vi "Write SP.vi"(8 "error in (no error)":errorcluster, 10 "SP":dbl, 11 "Y_H in":refnum<class "Y_H.lvclass">) -> (0 "error out":errorcluster, 3 "Y_H out":refnum<class "Y_H.lvclass">)   [LabVIEW 2019, in "Y_H.lvclass"]
uses:
  Y_H.lvclass
  Y_H.lvclass/Y_H.ctl
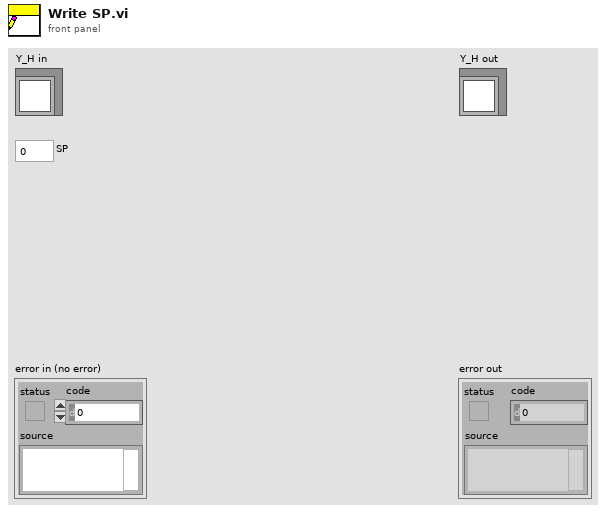
[diagram p1: front panel]
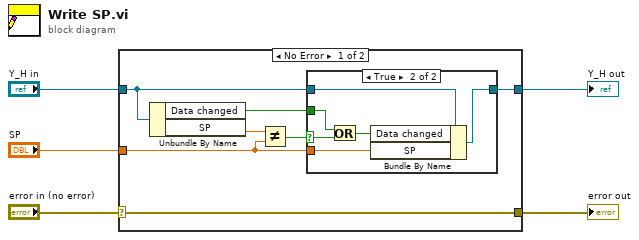
[diagram p0: block diagram]
diagram:
  n1 = case shown="No Error" "error in (no error)" {
    selector: "error in (no error)" -> [w12 w20]
    tunnel: [w12 w20] -> w1
    tunnel: [w11 w21] -> w2
    tunnel: "Y_H in" -> [w10 w21]
    tunnel: "SP" -> [w8 _]
    frame No Error {
      n2 = Unbundle By Name(w10) -> ("Data changed"=w6:bool, "SP"=w9:dbl)
      n3 = Not Equal?(x=w9, y=w8) -> (x != y?=w7:bool)
      n4 = case shown="True" w7 {
        selector: w7 -> [_ w16]
        tunnel: [w13 w19] -> w11
        tunnel: w10 -> [w13 w18]
        tunnel: w8 -> [_ w17]
        tunnel: w6 -> [_ w14]
        frame False {
        }
        frame True {
          n5 = Or(x=w14, y=w16) -> (x .or. y?=w15:bool)
          n6 = Bundle By Name(cluster=w18, "Data changed"=w15, "SP"=w17) -> (w19:refnum<class "Y_H.lvclass">)
        }
      }
    }
    frame Error {
    }
  }
  "error out" <- w1
  "Y_H out" <- w2
